vi "Polar Plot - PG Angle line.vi"(8 "grid measurements":T1 {"end angle" format="%0.2f"; "start angle" format="%0.2f"; "scale factors"."b" format="%0.2f"; "scale factors"."a" format="%0.2f"}, 9 "decade specs":cluster{"radius":i16, "label":string}[](array[cluster]), 11 "picture":picture) -> (3 "new picture":picture)   [LabVIEW 2020]
panel:
  in  "?":cluster{"angle":dbl, "min radius":i16}[](array[cluster])=[{"angle"=0.0, "min radius"=0}, {"angle"=15.0, "min radius"=25}, {"angle"=30.0, "min radius"=25}, {"angle"=45.0, "min radius"=10}, {"angle"=60.0, "min radius"=25}, {"angle"=75.0, "min radius"=25}] {"angle" format="%0.2f"}
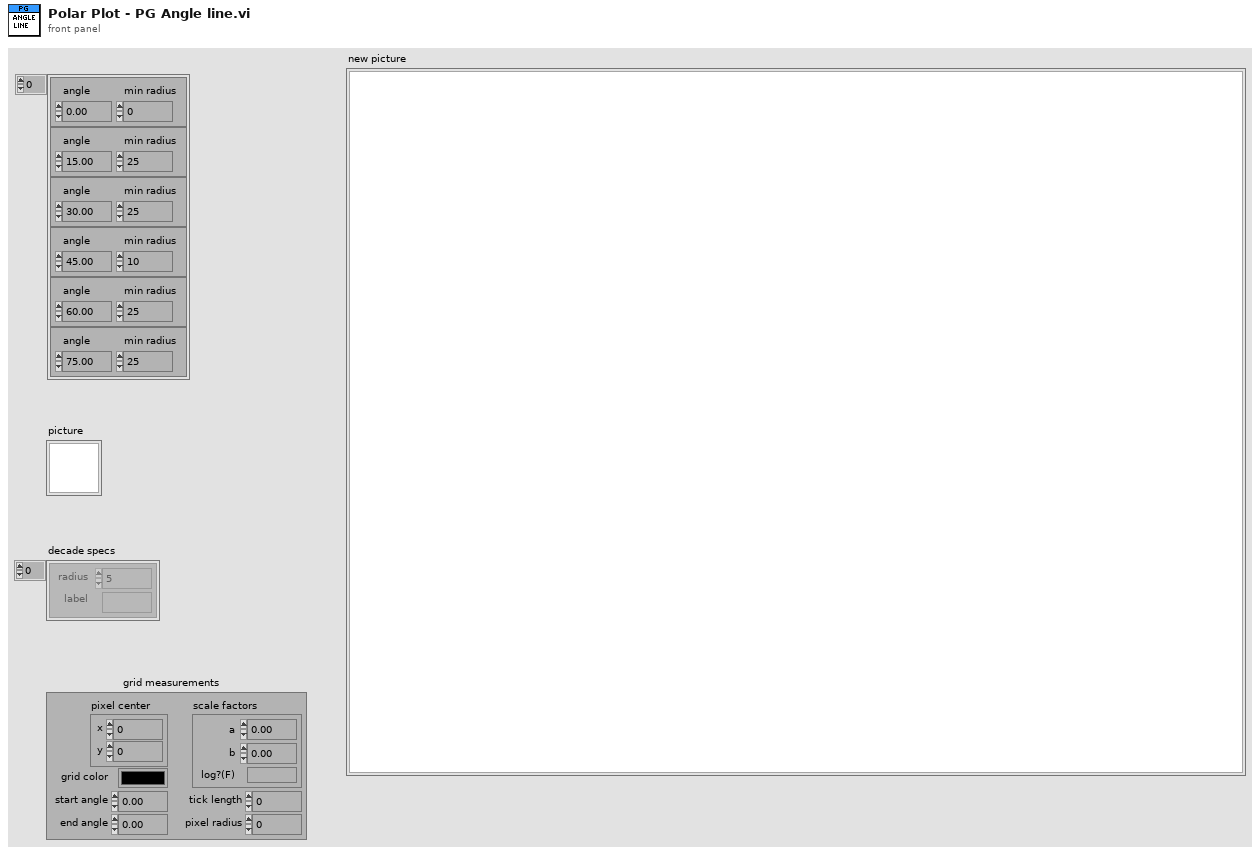
[diagram p1: front panel]
types:
  T1 = cluster{"pixel center":cluster{"x":i16, "y":i16}, "scale factors":cluster{"a":dbl, "b":dbl, "log?(F)":bool}, "grid color":u32, "start angle":dbl, "end angle":dbl, "tick length":i16, "pixel radius":i32}
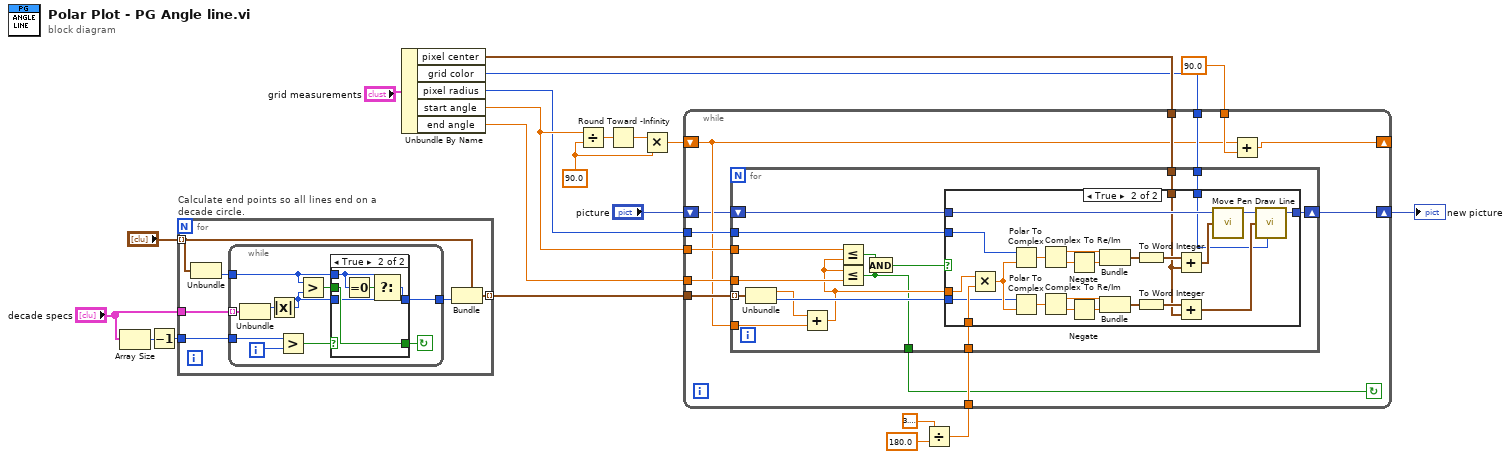
[diagram p0: block diagram]
diagram:
  w1 = 90.0
  n1 = Array Size(array="decade specs") -> (size(s)=w18:i32)
  n2 = Decrement(x=w18) -> (x-1=w16:i32)
  n3 = for "Calculate end points so all lines end on a decade circle." {
    tunnel: "?" -> [w24] mode=indexing
    tunnel: "decade specs" -> [w27]
    tunnel: w16 -> [w26]
    tunnel: [w22] -> w6 mode=indexing
    n4 = Unbundle(w24) -> ("min radius"=w25:i16)  [unwired: 1 out]
    n5 = while {
      tunnel: [w30] -> w23
      tunnel: w25 -> [w29]
      tunnel: w26 -> [w35]
      tunnel: w27 -> [w37] mode=indexing
      i -> [w36]
      stop <- w33 continue-if-true
      n6 = Unbundle(w37) -> ("radius"=w32:i16)  [unwired: 1 out]
      n7 = Absolute Value(x=w32) -> (abs(x)=w28:i16)
      n8 = Greater?(x=w35, y=w36) -> (0:w34:bool)
      n9 = Greater?(x=w29, y=w28) -> (0:w31:bool)
      n10 = case shown="True" w34 {
        selector: w34 -> [w39 _]
        tunnel: [w39 w44] -> w33
        tunnel: w28 -> [w38 w40]
        tunnel: w31 -> [_ w44]
        tunnel: [w38 w41] -> w30
        tunnel: w29 -> [_ w42]
        frame False {
          # "last element"
        }
        frame True {
          n11 = Equal To 0?(x=w42) -> (x = 0?=w43:bool)
          n12 = Select(t=w42, s=w43, f=w40) -> (s? t:f=w41:i16)
        }
      }
    }
    n13 = Bundle(cluster=w24, "min radius"=w23) -> (w22:cluster{"angle":dbl, "min radius":i16})  [unwired: 1 in]
  }
  n14 = Unbundle By Name("grid measurements") -> ("pixel center"=w20:cluster{"x":i16, "y":i16}, "grid color"=w5:u32, "pixel radius"=w7:i32, "start angle"=w9:dbl, "end angle"=w8:dbl)
  n15 = Divide(x=w9, y=w1) -> (x/y=w13:dbl)
  n16 = Round Toward -Infinity(1:w13) -> (0:w12:dbl)
  n17 = Multiply(x=w12, y=w1) -> (x*y=w11:dbl)
  n18 = Divide(x=3.141592653589793, y=180.0) -> (x/y=w10:dbl)
  n19 = while {
    shift-left: "picture" -> [w46]
    shift-right: [w45] -> w3
    tunnel: 90.0 -> [w49]
    tunnel: w5 -> [w50]
    tunnel: w20 -> [w51]
    tunnel: w6 -> [w52]
    tunnel: w7 -> [w53]
    tunnel: w8 -> [w54]
    tunnel: w9 -> [w55]
    tunnel: w10 -> [w56]
    shift-left: w11 -> [w48]
    shift-right: [w57] -> _
    stop <- w47 continue-if-true
    n20 = for {
      tunnel: w52 -> [w73] mode=indexing
      shift-right: [w71] -> w45
      shift-left: w46 -> [w72]
      tunnel: w51 -> [w70]
      tunnel: w50 -> [w69]
      tunnel: w56 -> [w68]
      tunnel: w55 -> [w64]
      tunnel: w54 -> [w63]
      tunnel: w53 -> [w62]
      tunnel: w48 -> [w61]
      tunnel: [w58] -> w47
      n21 = Unbundle(w73) -> ("angle"=w59:dbl, "min radius"=w67:i16)
      n22 = Add(x=w59, y=w61) -> (x+y=w60:dbl)
      n23 = Less Or Equal?(x=w64, y=w60) -> (x <= y?=w66:bool)
      n24 = Less Or Equal?(x=w60, y=w63) -> (x <= y?=w58:bool)
      n25 = And(x=w66, y=w58) -> (x .and. y?=w65:bool)
      n26 = case shown="True" w65 {
        tunnel: w72 -> [w74 w84]
        tunnel: [w74 w83] -> w71
        tunnel: w70 -> [_ w82]
        tunnel: w69 -> [_ w81]
        tunnel: w62 -> [_ w80]
        tunnel: w68 -> [_ w79]
        tunnel: w67 -> [_ w78]
        tunnel: w60 -> [_ w77]
        frame False {
        }
        frame True {
          n27 = Multiply(x=w77, y=w79) -> (x*y=w91:dbl)
          n28 = Polar To Complex(1:w91, 2:w80) -> (0:w90:cdb)
          n29 = Polar To Complex(1:w91, 2:w78) -> (0:w87:cdb)
          n30 = Complex To Re/Im(x + iy=w90) -> (x=w92:dbl, y=w93:dbl)
          n31 = Complex To Re/Im(x + iy=w87) -> (x=w88:dbl, y=w89:dbl)
          n32 = Negate(x=w93) -> (-x=w75:dbl)
          n33 = Negate(x=w89) -> (-x=w76:dbl)
          n34 = Bundle(w92, w75) -> (w85:cluster{dbl, dbl})  [unwired: 1 in]
          n35 = Bundle(w88, w76) -> (w86:cluster{dbl, dbl})  [unwired: 1 in]
          n36 = To Word Integer(number=w85) -> (16bit integer=w95:cluster{i16, i16})
          n37 = To Word Integer(number=w86) -> (16bit integer=w94:cluster{i16, i16})
          n38 = Add(x=w95, y=w82) -> (x+y=w97:cluster{i16, i16})
          n39 = Add(x=w94, y=w82) -> (x+y=w98:cluster{i16, i16})
          n40 = call <vilib>:"Move Pen.vi"("new position"=w97, "picture"=w84) -> ("new picture"=w96:picture)  [unwired: 3 in]
          n41 = call <vilib>:"Draw Line.vi"("picture"=w96, "end point"=w98, "color(black)"=w81) -> ("new picture"=w83:picture)  [unwired: 6 in]
        }
      }
    }
    n42 = Add(x=w48, y=w49) -> (x+y=w57:dbl)
  }
  "new picture" <- w3
